vi "Find_Exchanges.vi"(8 "error in (no error)":errorcluster caption="entrée d'erreur (pas d'erreur)", 9 "Type":T1, 10 "To_be_Found":string, 11 "Portfolio en entrée":refnum<class "Portfolio.lvclass"> caption="DNL_LabVIEW Object in") -> (0 "error out":errorcluster caption="sortie d'erreur", 1 "Gain/loss":dbl, 2 "Found ?":bool, 3 "Portfolio en sortie":refnum<class "Portfolio.lvclass"> caption="DNL_LabVIEW Object out")   [LabVIEW 2012, in "Portfolio.lvclass"]
uses:
  Portfolio.lvclass
  Find_Exchanges.ctl
  Portfolio.lvclass/Portfolio.ctl
  Exchanges/Exchanges.lvclass
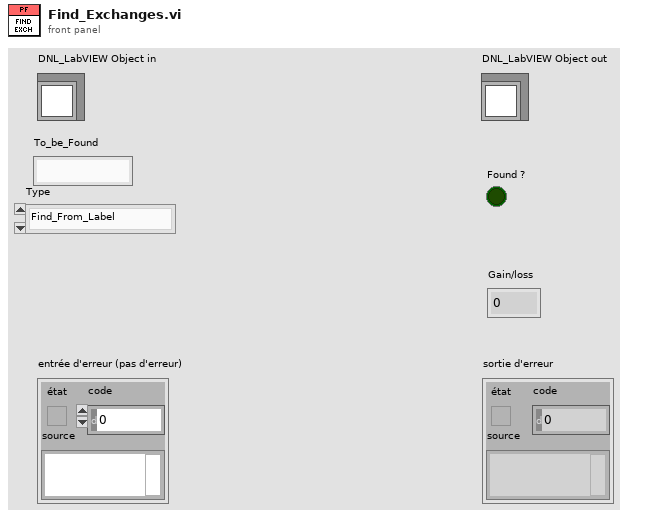
[diagram p1: front panel]
types:
  T1 = typedef "Find_Exchanges.ctl" = enum16{"Find_From_Label", "Find_From_ISIN"}
  T2 = typedef "Exchange Parameters.ctl" = cluster{"Date":timestamp, "Exchange Type":T3, "ISIN":string, "Label":string, "Price":dbl, "Qty":dbl, "Currency":T4, "Tax":dbl, "Comment":string, "PRU":dbl}
  T3 = typedef "Exchange.lvclass/Exchange Type Enum.ctl" = enum16{"ACHAT", "VENTE"}
  T4 = typedef "Currencies.ctl" = enum16{"Euro", "Dollar", "Yen", "RIM", "CHF"}
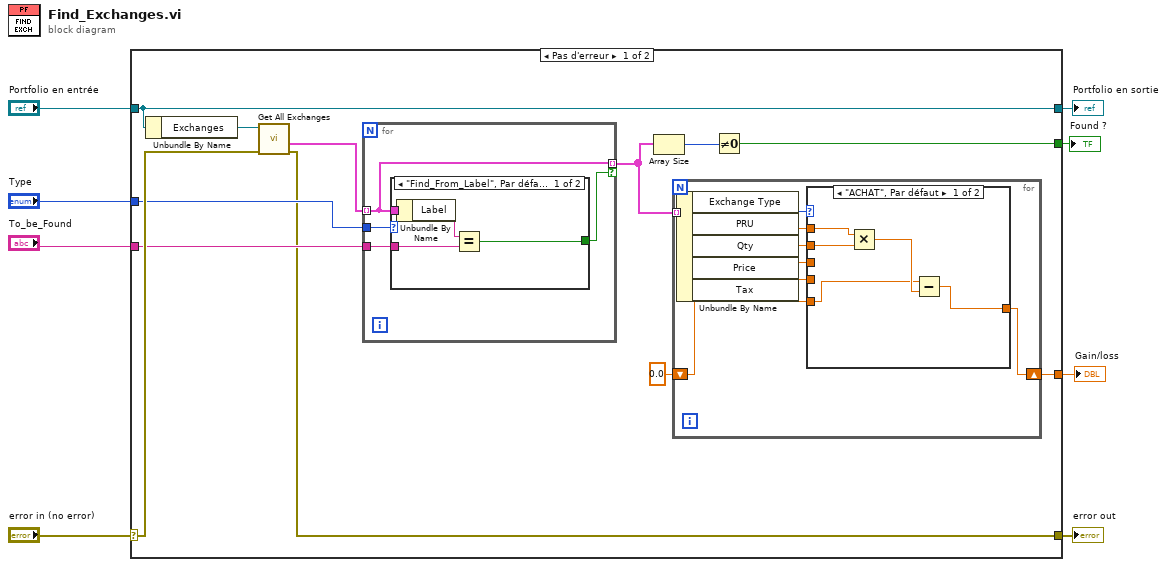
[diagram p0: block diagram]
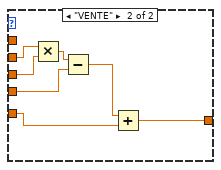
[diagram p2: hidden frame]
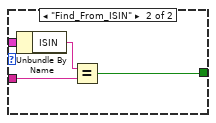
[diagram p3: hidden frame]
diagram:
  n1 = case shown="Pas d'erreur" "error in (no error)" {
    selector: "error in (no error)" -> [w19 w54]
    tunnel: [w9 w54] -> w7
    tunnel: [w20 w53] -> w5
    tunnel: "Portfolio en entrée" -> [w20 w53]
    tunnel: "To_be_Found" -> [w16 _]
    tunnel: "Type" -> [w15 _]
    tunnel: [w13 _] -> w2
    tunnel: [w10 _] -> w1
    frame No Error {
      n2 = Unbundle By Name(w20) -> ("Exchanges"=w18:refnum<class "Exchanges.lvclass">)
      n3 = call "Get All Exchanges.vi"("error in (no error)"=w19, "Exchanges en entrée"=w18) -> ("error out"=w9:errorcluster, "Exchanges"=w17:T2[])  [unwired: 5 in, 3 out]
      n4 = for {
        tunnel: w17 -> [w44] mode=indexing
        tunnel: [w44] -> w12 mode=indexing if=w42
        tunnel: w16 -> [w43]
        tunnel: w15 -> [w41]
        n5 = case shown="\"Find_From_Label\", Par défaut" w41 {
          tunnel: w44 -> [w48 w52]
          tunnel: w43 -> [w46 w50]
          tunnel: [w45 w49] -> w42
          frame "Find_From_Label", Default {
            n6 = Unbundle By Name(w48) -> ("Label"=w47:string)
            n7 = Equal?(x=w47, y=w46) -> (x = y?=w45:bool)
          }
          frame "Find_From_ISIN" {
            n8 = Unbundle By Name(w52) -> ("ISIN"=w51:string)
            n9 = Equal?(x=w51, y=w50) -> (x = y?=w49:bool)
          }
        }
      }
      n10 = Array Size(array=w12) -> (size(s)=w14:i32)
      n11 = for {
        tunnel: w12 -> [w28] mode=indexing
        shift-right: [w23] -> w10
        shift-left: 0.0 -> [w22]
        n12 = Unbundle By Name(w28) -> ("Exchange Type"=w27:T3, "PRU"=w26:dbl, "Qty"=w25:dbl, "Price"=w24:dbl, "Tax"=w21:dbl)
        n13 = case shown="\"ACHAT\", Par défaut" w27 {
          tunnel: w26 -> [w32 _]
          tunnel: w25 -> [w33 w40]
          tunnel: w24 -> [_ w39]
          tunnel: [w29 w34] -> w23
          tunnel: w22 -> [w30 w35]
          tunnel: w21 -> [_ w37]
          frame "ACHAT", Default {
            n14 = Multiply(x=w32, y=w33) -> (x*y=w31:dbl)
            n15 = Subtract(x=w30, y=w31) -> (x-y=w29:dbl)
          }
          frame "VENTE" {
            n16 = Multiply(x=w40, y=w39) -> (x*y=w38:dbl)
            n17 = Subtract(x=w38, y=w37) -> (x-y=w36:dbl)
            n18 = Add(x=w36, y=w35) -> (x+y=w34:dbl)
          }
        }
      }
      n19 = Not Equal To 0?(x=w14) -> (x != 0?=w13:bool)
    }
    frame Error {
    }
  }
  "error out" <- w7
  "Portfolio en sortie" <- w5
  "Found ?" <- w2
  "Gain/loss" <- w1
